vi "Solve1.vi"(8 "Error In":errorcluster, 11 "object in":refnum<class "2022_2.lvclass">) -> (0 "Error Out":errorcluster, 2 "Result":u64, 3 "object out":refnum<class "2022_2.lvclass">)   [LabVIEW 2020, in "2022_2.lvclass"]
uses:
  2022_2.lvclass
  2022_2.lvclass/2022_2.ctl
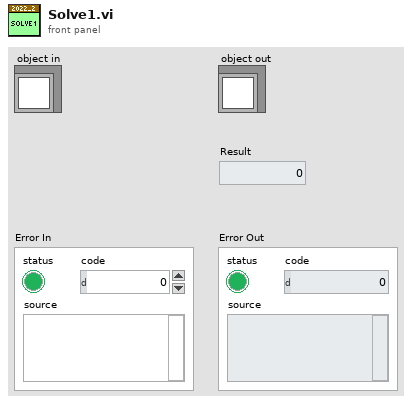
[diagram p1: front panel]
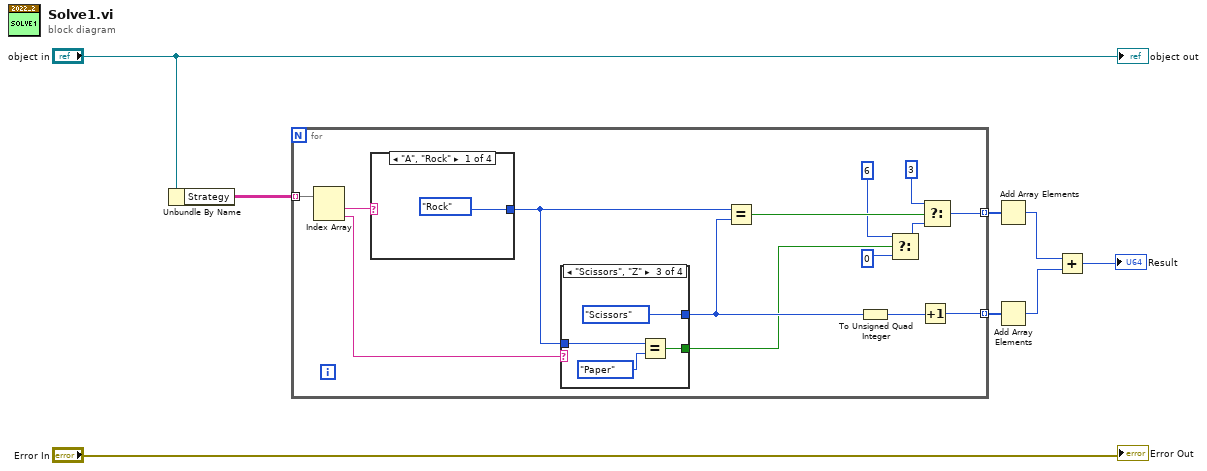
[diagram p0: block diagram]
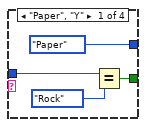
[diagram p2: hidden frame]
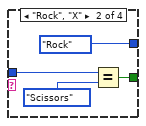
[diagram p3: hidden frame]
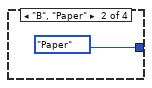
[diagram p5: hidden frame]
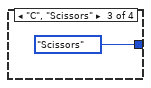
[diagram p6: hidden frame]
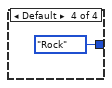
[diagram p7: hidden frame]
diagram:
  n1 = Unbundle By Name("object in") -> ("Strategy"=w5:string[][])
  n2 = for {
    tunnel: w5 -> [w22] mode=indexing
    tunnel: [w15] -> w4 mode=indexing
    tunnel: [w12] -> w2 mode=indexing
    n3 = Index Array(array=w22) -> (element #1=w21:string, element #2=w20:string)  [unwired: 2 in]
    n4 = case shown="\"A\", \"Rock\"" w21 {
      tunnel: [enum16{"Rock", "Paper", "Scissors"}."Rock" enum16{"Rock", "Paper", "Scissors"}."Paper" enum16{"Rock", "Paper", "Scissors"}."Scissors" enum16{"Rock", "Paper", "Scissors"}."Rock"] -> w9
      frame "A", "Rock" {
      }
      frame "B", "Paper" {
      }
      frame "C", "Scissors" {
      }
      frame Default {
      }
    }
    n5 = case shown="\"Scissors\", \"Z\"" w20 {
      tunnel: [enum16{"Rock", "Paper", "Scissors"}."Paper" enum16{"Rock", "Paper", "Scissors"}."Rock" enum16{"Rock", "Paper", "Scissors"}."Scissors" _] -> w14
      tunnel: [w23 w27 w31 _] -> w11
      tunnel: w9 -> [w24 w29 w32 _]
      frame "Paper", "Y" {
        n6 = Equal?(x=w24, y=enum16{"Rock", "Paper", "Scissors"}."Rock") -> (x = y?=w23:bool)
      }
      frame "Rock", "X" {
        n7 = Equal?(x=w29, y=enum16{"Rock", "Paper", "Scissors"}."Scissors") -> (x = y?=w27:bool)
      }
      frame "Scissors", "Z" {
        n8 = Equal?(x=w32, y=enum16{"Rock", "Paper", "Scissors"}."Paper") -> (x = y?=w31:bool)
      }
      frame Default {
      }
    }
    n9 = Equal?(x=w9, y=w14) -> (x = y?=w19:bool)
    n10 = To Unsigned Quad Integer(1:w14) -> (0:w13:u64)
    n11 = Select(t=u64 6, s=w11, f=u64 0) -> (s? t:f=w16:u64)
    n12 = Increment(x=w13) -> (x+1=w12:u64)
    n13 = Select(t=u64 3, s=w19, f=w16) -> (s? t:f=w15:u64)
  }
  n14 = Add Array Elements(numeric array=w4) -> (sum=w3:u64)
  n15 = Add Array Elements(numeric array=w2) -> (sum=w1:u64)
  n16 = Add(x=w3, y=w1) -> (x+y=→"Result":u64)
  "Error Out" <- "Error In"
  "object out" <- "object in"
